vi "Remove Section.vi"(7 "Section Name":string, 8 "error in (no error)":errorcluster, 11 "Config in":T1) -> (0 "error out":errorcluster, 2 "Section Found?":bool, 3 "Config out":T1)   [LabVIEW 2022 SP3, in "LabVIEW-Config.lvlib"]
uses:
  LabVIEW-Config.lvlib
  Config.ctl
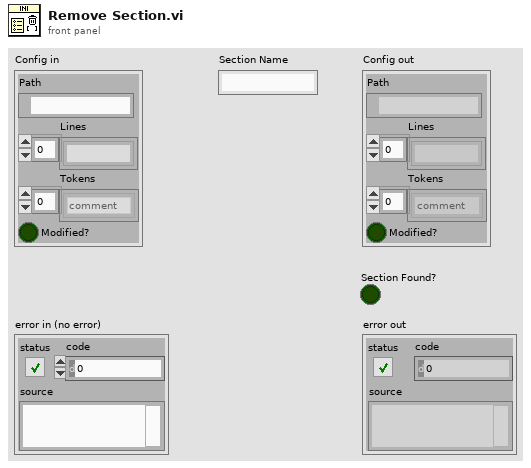
[diagram p1: front panel]
types:
  T1 = typedef "LabVIEW-Config.lvlib/Config.ctl" = cluster{"Path":path, "Lines":string[], "Tokens":enum8{"comment", "section", "key"}[], "Modified?":bool}
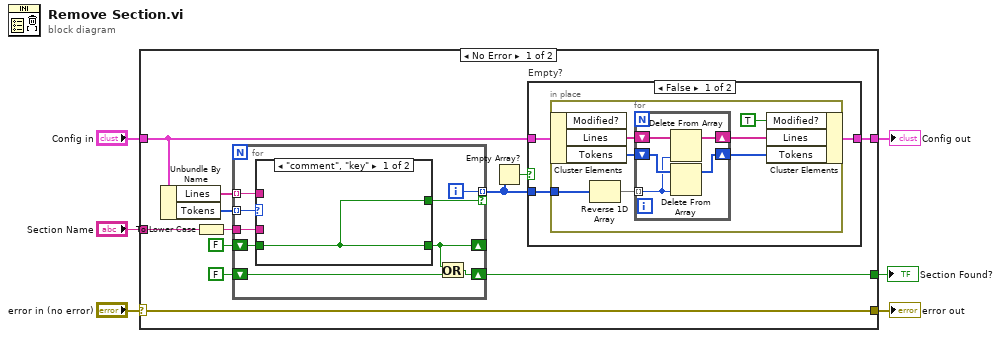
[diagram p0: block diagram]
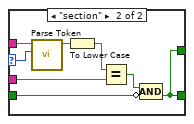
[diagram p2: hidden frame]
diagram:
  n1 = case shown="No Error" "error in (no error)" {
    selector: "error in (no error)" -> [w16 w54]
    tunnel: "Config in" -> [w9 w53]
    tunnel: [w16 w54] -> w5
    tunnel: [w10 w53] -> w3
    tunnel: "Section Name" -> [w15 _]
    tunnel: [w11 _] -> w1
    frame No Error {
      n2 = Unbundle By Name(w9) -> ("Lines"=w17:string[], "Tokens"=w18:enum8{"comment", "section", "key"}[])
      n3 = To Lower Case(string=w15) -> (all lower case string=w14:string)
      n4 = for {
        tunnel: w18 -> [w27] mode=indexing
        tunnel: w17 -> [w26] mode=indexing
        tunnel: [w19] -> w8 mode=indexing if=w23
        tunnel: w14 -> [w25]
        shift-right: [w22] -> _
        shift-left: FALSE -> [w24]
        shift-right: [w21] -> w11
        shift-left: FALSE -> [w20]
        i -> [w19]
        n5 = case shown="\"comment\", \"key\"" w27 {
          selector: w27 -> [_ w30]
          tunnel: w26 -> [_ w31]
          tunnel: w25 -> [_ w36]
          tunnel: [w28 w32] -> w22
          tunnel: w24 -> [w28 w34]
          tunnel: [w28 w32] -> w23
          frame "comment", "key" {
          }
          frame "section" {
            n6 = call "Parse Token.vi"("Token"=w30, "Line"=w31) -> ("Name"=w29:string)  [unwired: 8 in, 1 out]
            n7 = To Lower Case(string=w29) -> (all lower case string=w35:string)
            n8 = Equal?(x=w35, y=w36) -> (x = y?=w33:bool)
            n9 = Compound Arithmetic op=AND(w33, invert w34) -> (w32:bool)
          }
        }
        n10 = Or(x=w22, y=w20) -> (x .or. y?=w21:bool)
      }
      n11 = Empty Array?(array=w8) -> (empty?=w7:bool)
      n12 = case "Empty?" shown="False" w7 {
        tunnel: [w39 w52] -> w10
        tunnel: w9 -> [w38 w52]
        tunnel: w8 -> [w37 _]
        frame False {
          n13 = in-place {
            in-place-border: w37 -> [w45]
            n14 = in-place-cluster #1(w38) -> ("Lines"=w44:string[], "Tokens"=w43:enum8{"comment", "section", "key"}[])  [unwired: 1 out]
            n15 = Reverse 1D Array(array=w45) -> (reversed array=w40:i32[])
            n16 = for {
              shift-right: [w50] -> w41
              shift-left: w44 -> [w51]
              shift-right: [w47] -> w42
              shift-left: w43 -> [w49]
              tunnel: w40 -> [w48] mode=indexing
              n17 = Delete From Array(array=w51, index=w48) -> (array with subset deleted=w50:string[])  [unwired: 1 in, 1 out]
              n18 = Delete From Array(array=w49, index=w48) -> (array with subset deleted=w47:enum8{"comment", "section", "key"}[])  [unwired: 1 in, 1 out]
            }
            n19 = in-place-cluster #1("Modified?"=TRUE, "Lines"=w41, "Tokens"=w42) -> (w39:T1)
          }
        }
        frame True {
        }
      }
    }
    frame Error {
    }
  }
  "error out" <- w5
  "Config out" <- w3
  "Section Found?" <- w1
